vi "welcome.vi"() -> ()   [LabVIEW 2017]
uses:
  GLOBAL/auto.vi
  GLOBAL/all vi close.vi
panel:
  out "first time direct auto":bool
  in  "error in":errorcluster
  in  "EXIT":bool
  in  "PRINTER":bool
  in  "DATA\nHISTORY":bool
  in  "MAIN":bool
  in  "LOGOUT":bool
  in  "USER":bool
  in  "COUNTER":bool
  in  "SETTING":bool
  in  "SHIFT SETTING":bool
  in  "LOGIN":bool
  # "TRACEABILITY"
  # "Powered By- NI Vision, Pune"
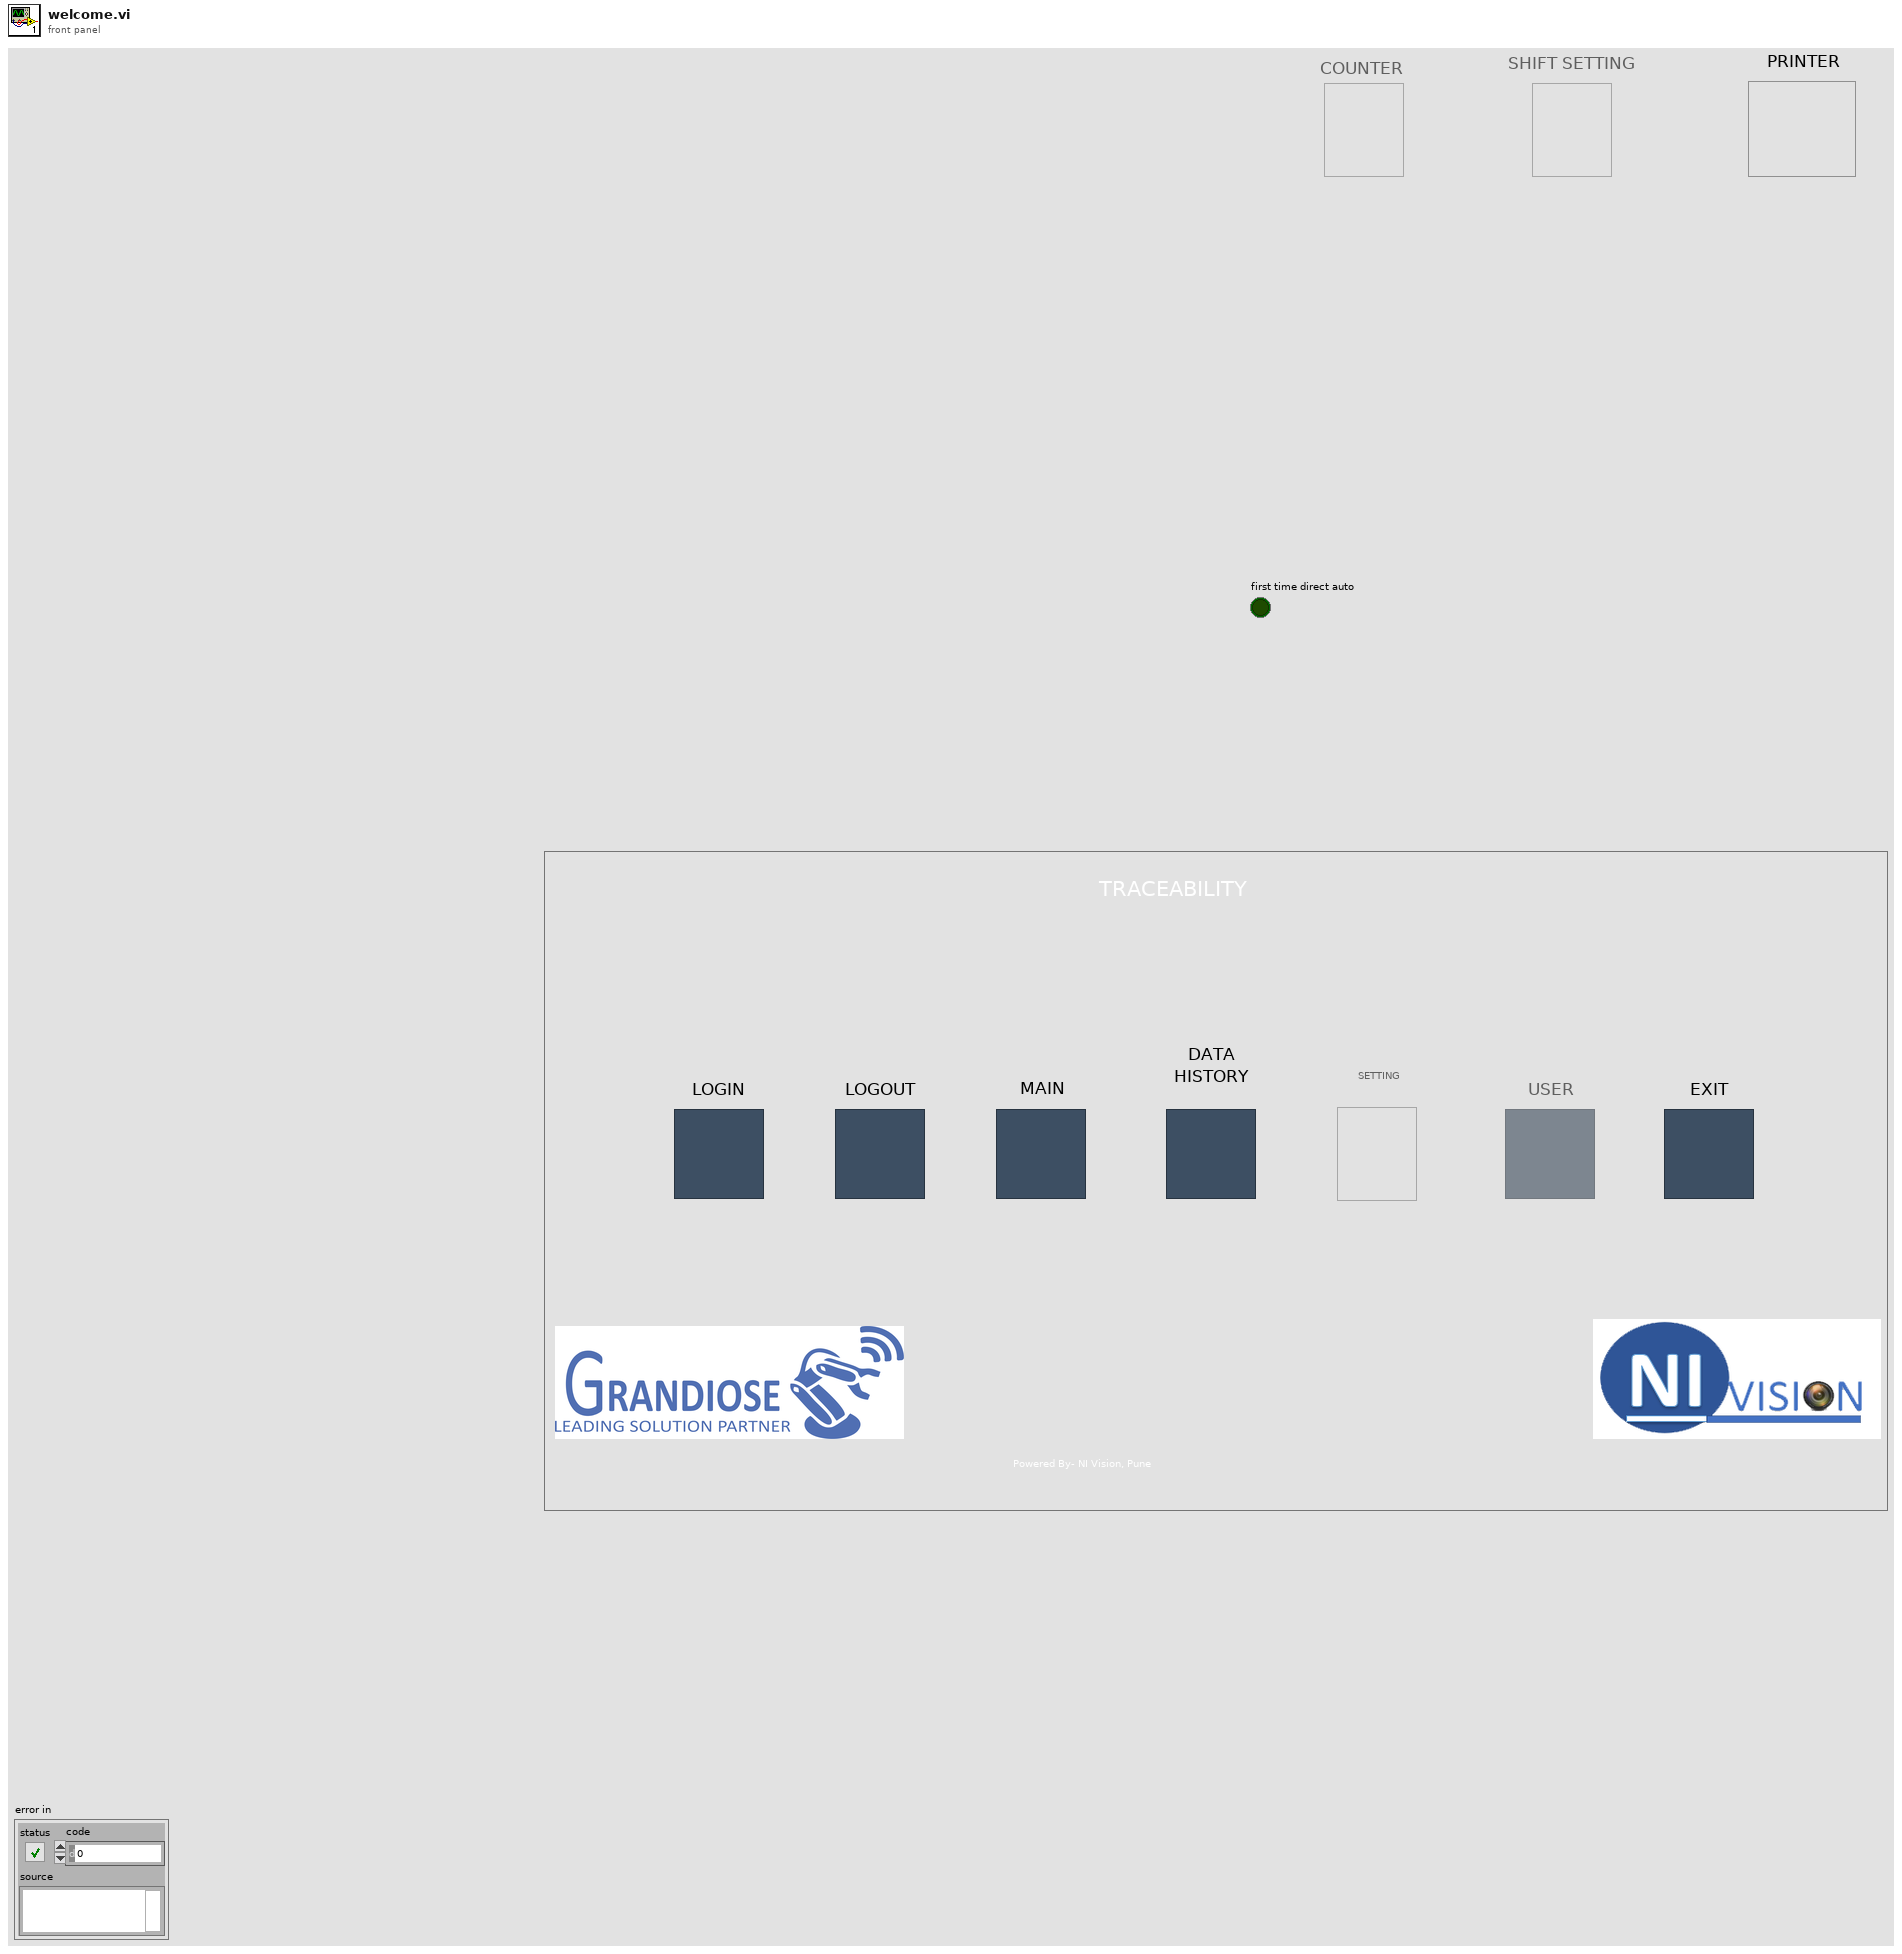
[diagram p1: front panel]
types:
  T1 = enum8{"Enabled", "Disabled", "Disabled and Grayed Out"}
  T2 = enum32{"Invalid", "Standard", "Closed", "Hidden", "Minimized", "Maximized"}
  T3 = enum32{"invalid app kind", "Development System", "Run Time System", "Student Edition", "Embedded LabVIEW", "Evaluation", "Custom"}
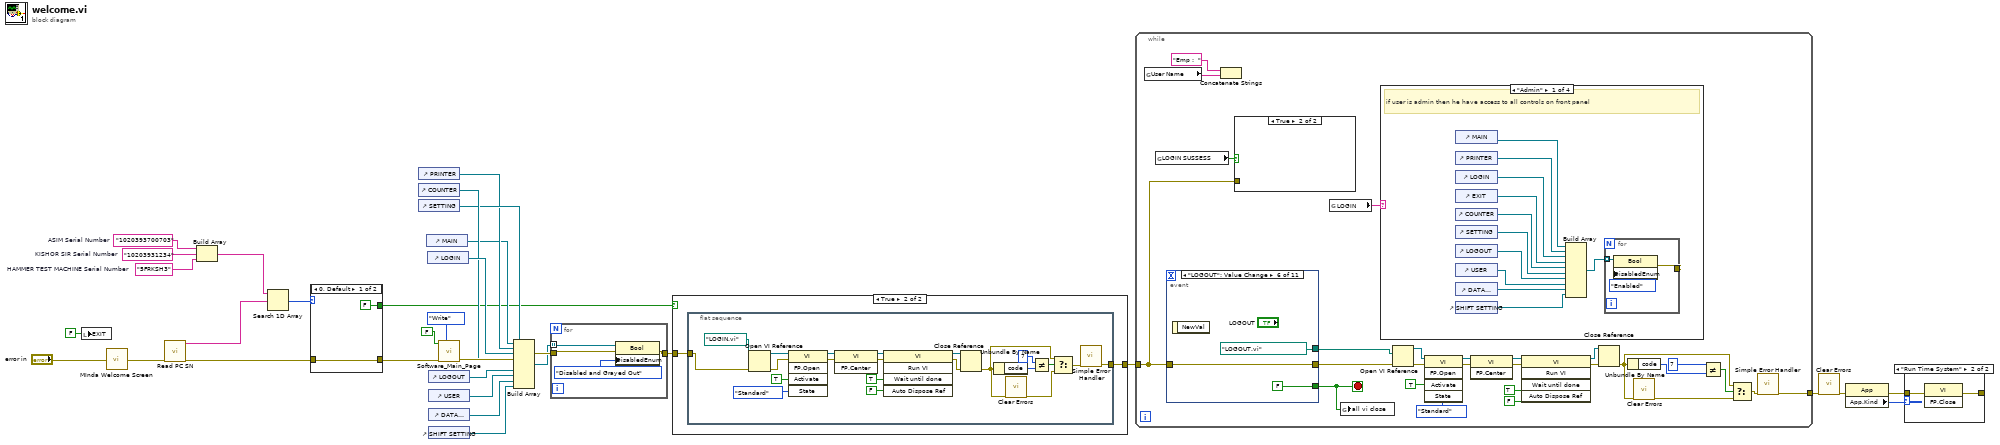
[diagram p0: block diagram]
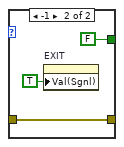
[diagram p3: hidden frame]
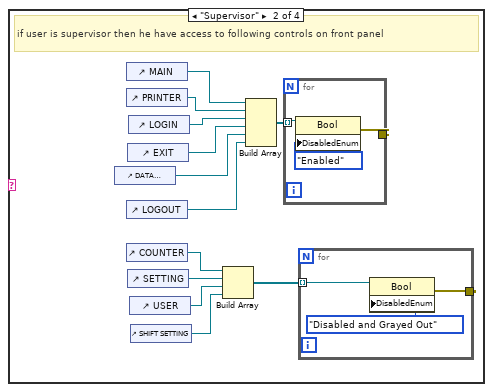
[diagram p6: hidden frame]
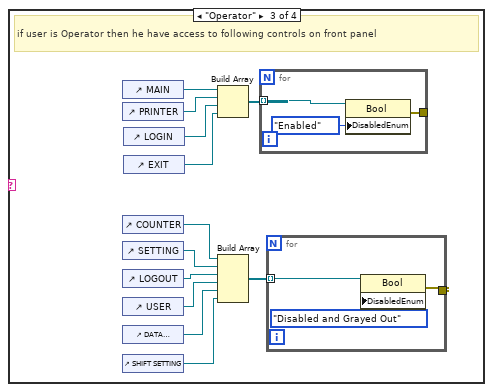
[diagram p7: hidden frame]
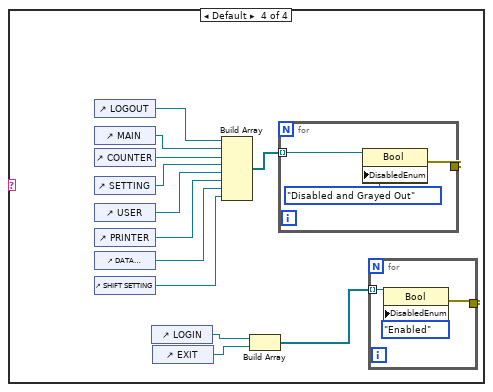
[diagram p8: hidden frame]
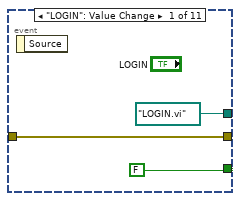
[diagram p9: hidden frame]
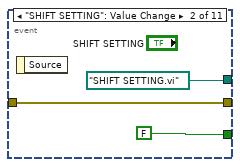
[diagram p10: hidden frame]
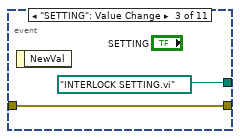
[diagram p11: hidden frame]
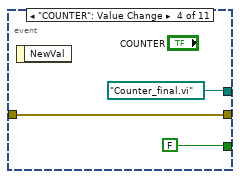
[diagram p12: hidden frame]
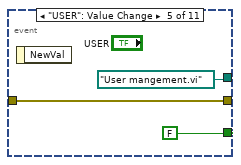
[diagram p13: hidden frame]
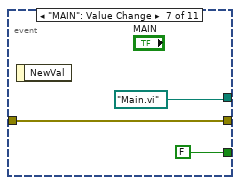
[diagram p14: hidden frame]
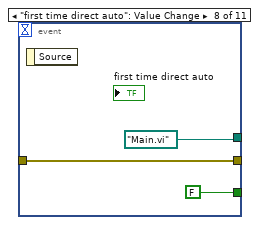
[diagram p15: hidden frame]
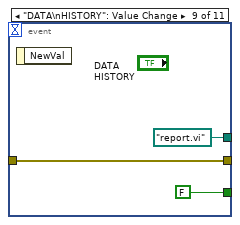
[diagram p16: hidden frame]
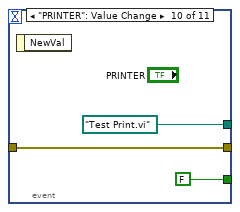
[diagram p17: hidden frame]
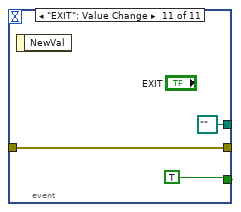
[diagram p18: hidden frame]
diagram:
  w6 = "5FRKSH3"  # HAMMER TEST MACHINE Serial Number
  w7 = "10203931234"  # KISHOR SIR Serial Number
  w8 = "1020393700703"  # ASIM Serial Number
  n1 = local write "EXIT"(FALSE) -> ()
  n2 = call "MInda Welcome Screen.vi"("error in"="error in") -> ("error out"=w10:errorcluster)
  n3 = call "Read PC SN.vi"("error in (no error)"=w10) -> ("error out"=w3:errorcluster, "Serial Number"=w9:string)  [unwired: 9 in]
  n4 = Build Array(w8, w7, w6) -> (w5:string[])
  n5 = Search 1D Array(1D array=w5, element=w9) -> (index of element=w4:i32)  [unwired: 1 in]
  n6 = case shown="0, Default" w4 {
    tunnel: [w33 w35] -> w2
    tunnel: w3 -> [w33 w35]
    tunnel: [FALSE FALSE] -> w1
    frame 0, Default {
    }
    frame -1 {
      n7 = property on="EXIT" class="Bool (strict)"("Val(Sgnl)"=TRUE) -> ()  [unwired: 2 in, 2 out]
    }
  }
  n8 = control-ref of="PRINTER"() -> (w14:refnum<vi>)
  n9 = control-ref of="COUNTER"() -> (w20:refnum<vi>)
  n10 = control-ref of="SETTING"() -> (w19:refnum<vi>)
  n11 = control-ref of="MAIN"() -> (w13:refnum<vi>)
  n12 = control-ref of="LOGIN"() -> (w21:refnum<vi>)
  n13 = control-ref of="LOGOUT"() -> (w18:refnum<vi>)
  n14 = control-ref of="USER"() -> (w17:refnum<vi>)
  n15 = control-ref of="DATA\nHISTORY"() -> (w16:refnum<vi>)
  n16 = control-ref of="SHIFT SETTING"() -> (w15:refnum<vi>)
  n17 = call "Software_Main_Page.vi"("Enum"=enum16{"Read", "Write"}."Write", "error in (no error)"=w2, "Main_Page_in"=FALSE) -> ("error out"=w23:errorcluster)  [unwired: 7 in, 1 out]
  n18 = Build Array(w13, w14, w21, w20, w19, w18, w17, w16, w15) -> (w22:refnum<vi>[])
  n19 = for {
    tunnel: w22 -> [w40] mode=indexing
    tunnel: w23 -> [w38]
    tunnel: [w37] -> w12
    n20 = property class="Bool"(reference=w40, error in=w38, "DisabledEnum"=T1."Disabled and Grayed Out" ("Disabled")) -> (error out=w37:errorcluster)  [unwired: 1 out]
  }
  n21 = case shown="True" w1 {
    tunnel: [w41 w43] -> w30
    tunnel: w12 -> [w41 w42]
    frame False {
    }
    frame True {
      n22 = flat-sequence {
        tunnel: [w45] -> w43
        tunnel: w42 -> [w44]
        frame #0 {
          n23 = Open VI Reference(vi path=path "LOGIN.vi", error in (no error)=w44) -> (vi reference=w52:refnum<vi>, error out=w64:errorcluster)  [unwired: 4 in]
          n24 = invoke class="VI" method="FP.Open"(reference=w52, error in=w64, "Activate"=TRUE ("Activate?"), "State"=T2."Standard") -> (reference out=w63:refnum<vi>, error out=w58:errorcluster)  [unwired: 1 in, 3 out]
          n25 = invoke class="VI" method="FP.Center"(reference=w63, error in=w58) -> (reference out=w59:refnum<vi>, error out=w60:errorcluster)  [unwired: 1 in, 1 out]
          n26 = invoke class="VI" method="Run VI"(reference=w59, error in=w60, "Wait until done"=TRUE ("Wait Until Done"), "Auto Dispose Ref"=FALSE ("Auto Dispose Reference")) -> (reference out=w61:refnum<vi>, error out=w62:errorcluster)  [unwired: 1 in, 3 out]
          n27 = Close Reference(reference=w61, error in (no error)=w62) -> (error out=w53:errorcluster)
          n28 = Unbundle By Name(w53) -> ("code"=w57:i32)
          n29 = call <vilib>:"Clear Errors.vi"("error in (no error)"=w53) -> ("error out"=w55:errorcluster)  [unwired: 5 in, 1 out]
          n30 = Not Equal?(x=7, y=w57) -> (x != y?=w56:bool)
          n31 = Select(t=w53, s=w56, f=w55) -> (s? t:f=w54:errorcluster)
          n32 = call <vilib>:"Simple Error Handler.vi"("error in (no error)"=w54) -> ("error out"=w45:errorcluster)  [unwired: 4 in, 4 out]
        }
      }
    }
  }
  n33 = while {
    tunnel: w30 -> [w67]
    tunnel: [w71] -> w31
    stop <- w69 stop-if-true
    n34 = global read "auto.vi" "User Name"() -> (w66:string)
    n35 = global read "auto.vi" "LOGIN SUSSESS"() -> (w68:bool)
    n36 = event shown="[5] \"LOGOUT\": Value Change" {
      selector: _ -> [_ _ _ _ _ _ _ _ _ _ _]
      dyn-events: _ -> [_ _ _ _ _ _ _ _ _ _ _]
      timeout: _ -> [_ _ _ _ _ _ _ _ _ _ _]
      tunnel: [FALSE FALSE _ FALSE FALSE FALSE FALSE FALSE FALSE FALSE TRUE] -> w69
      tunnel: [path "LOGIN.vi" ("vi path") path "SHIFT SETTING.vi" ("vi path") path "INTERLOCK SETTING.vi" ("vi path") path "Counter_final.vi" ("vi path") path "User mangement.vi" ("vi path") path "LOGOUT.vi" ("vi path") path "Main.vi" ("vi path") path "Main.vi" ("vi path") path "report.vi" ("vi path") path "Test Print.vi" ("vi path") path "" ("vi path")] -> w72
      tunnel: w67 -> [w161 w165 w167 w168 w171 w174 w178 w181 w183 w186 w190]
      tunnel: [w161 w165 w167 w168 w171 w174 w178 w181 w183 w186 w190] -> w73
      event "LOGIN": Value Change {
        n37 = event-data() -> ()  [unwired: 1 in, 1 out]
      }
      event "SHIFT SETTING": Value Change {
        n38 = event-data() -> ()  [unwired: 1 in, 1 out]
      }
      event "SETTING": Value Change {
        n39 = event-data() -> ()  [unwired: 1 in, 1 out]
      }
      event "COUNTER": Value Change {
        n40 = event-data() -> ()  [unwired: 1 in, 1 out]
      }
      event "USER": Value Change {
        n41 = event-data() -> ()  [unwired: 1 in, 1 out]
      }
      event "LOGOUT": Value Change {
        n42 = event-data() -> ()  [unwired: 1 in, 1 out]
      }
      event "MAIN": Value Change {
        n43 = event-data() -> ()  [unwired: 1 in, 1 out]
      }
      event "first time direct auto": Value Change {
        n44 = event-data() -> ()  [unwired: 1 in, 1 out]
      }
      event "DATA\nHISTORY": Value Change {
        n45 = event-data() -> ()  [unwired: 1 in, 1 out]
      }
      event "PRINTER": Value Change {
        n46 = event-data() -> ()  [unwired: 1 in, 1 out]
      }
      event "EXIT": Value Change {
        n47 = event-data() -> ()  [unwired: 1 in, 1 out]
      }
    }
    n48 = Concatenate Strings("Emp :  " ("string"), w66) -> ()  [unwired: 1 out]
    n49 = case shown="True" w68 {
      tunnel: w67 -> [_ _]
      frame False {
      }
      frame True {
      }
    }
    n50 = global read "auto.vi" "LOGIN"() -> (w70:string)
    n51 = global write "all vi close.vi" "all vi close"(w69) -> ()
    n52 = case shown="\"Admin\"" w70 {
      frame "Admin" {
        # "if user is admin then he have access to all controls on front panel"
        n53 = control-ref of="MAIN"() -> (w92:refnum<vi>)
        n54 = control-ref of="PRINTER"() -> (w93:refnum<vi>)
        n55 = control-ref of="LOGIN"() -> (w101:refnum<vi>)
        n56 = control-ref of="EXIT"() -> (w100:refnum<vi>)
        n57 = control-ref of="COUNTER"() -> (w99:refnum<vi>)
        n58 = control-ref of="SETTING"() -> (w98:refnum<vi>)
        n59 = control-ref of="LOGOUT"() -> (w97:refnum<vi>)
        n60 = control-ref of="USER"() -> (w96:refnum<vi>)
        n61 = control-ref of="DATA\nHISTORY"() -> (w95:refnum<vi>)
        n62 = control-ref of="SHIFT SETTING"() -> (w94:refnum<vi>)
        n63 = Build Array(w92, w93, w101, w100, w99, w98, w97, w96, w95, w94) -> (w102:refnum<vi>[])
        n64 = for {
          tunnel: w102 -> [w103] mode=indexing
          tunnel: [w104] -> _
          n65 = property class="Bool"(reference=w103, "DisabledEnum"=T1."Enabled" ("Disabled")) -> (error out=w104:errorcluster)  [unwired: 1 in, 1 out]
        }
      }
      frame "Supervisor" {
        # "if user is supervisor then he have access to following controls on front panel"
        n66 = control-ref of="DATA\nHISTORY"() -> (w113:refnum<vi>)
        n67 = control-ref of="MAIN"() -> (w106:refnum<vi>)
        n68 = control-ref of="PRINTER"() -> (w107:refnum<vi>)
        n69 = control-ref of="LOGOUT"() -> (w112:refnum<vi>)
        n70 = control-ref of="COUNTER"() -> (w111:refnum<vi>)
        n71 = control-ref of="EXIT"() -> (w114:refnum<vi>)
        n72 = control-ref of="SETTING"() -> (w110:refnum<vi>)
        n73 = control-ref of="LOGIN"() -> (w115:refnum<vi>)
        n74 = control-ref of="USER"() -> (w109:refnum<vi>)
        n75 = control-ref of="SHIFT SETTING"() -> (w108:refnum<vi>)
        n76 = Build Array(w111, w110, w109, w108) -> (w116:refnum<vi>[])
        n77 = Build Array(w106, w107, w115, w114, w113, w112) -> (w117:refnum<vi>[])
        n78 = for {
          tunnel: w117 -> [w121] mode=indexing
          tunnel: [w122] -> _
          n79 = property class="Bool"(reference=w121, "DisabledEnum"=T1."Enabled" ("Disabled")) -> (error out=w122:errorcluster)  [unwired: 1 in, 1 out]
        }
        n80 = for {
          tunnel: [w119] -> _
          tunnel: w116 -> [w118] mode=indexing
          n81 = property class="Bool"(reference=w118, "DisabledEnum"=T1."Disabled and Grayed Out" ("Disabled")) -> (error out=w119:errorcluster)  [unwired: 1 in, 1 out]
        }
      }
      frame "Operator" {
        # "if user is Operator then he have access to following controls on front panel"
        n82 = control-ref of="MAIN"() -> (w124:refnum<vi>)
        n83 = control-ref of="PRINTER"() -> (w133:refnum<vi>)
        n84 = control-ref of="COUNTER"() -> (w127:refnum<vi>)
        n85 = control-ref of="SETTING"() -> (w132:refnum<vi>)
        n86 = control-ref of="LOGOUT"() -> (w131:refnum<vi>)
        n87 = control-ref of="USER"() -> (w130:refnum<vi>)
        n88 = control-ref of="DATA\nHISTORY"() -> (w129:refnum<vi>)
        n89 = control-ref of="SHIFT SETTING"() -> (w128:refnum<vi>)
        n90 = control-ref of="LOGIN"() -> (w126:refnum<vi>)
        n91 = control-ref of="EXIT"() -> (w125:refnum<vi>)
        n92 = Build Array(w124, w133, w126, w125) -> (w135:refnum<vi>[])
        n93 = Build Array(w127, w132, w131, w130, w129, w128) -> (w134:refnum<vi>[])
        n94 = for {
          tunnel: w135 -> [w141] mode=indexing
          tunnel: [w139] -> _
          n95 = property class="Bool"(reference=w141, "DisabledEnum"=T1."Enabled" ("Disabled")) -> (error out=w139:errorcluster)  [unwired: 1 in, 1 out]
        }
        n96 = for {
          tunnel: w134 -> [w138] mode=indexing
          tunnel: [w136] -> _
          n97 = property class="Bool"(reference=w138, "DisabledEnum"=T1."Disabled and Grayed Out" ("Disabled")) -> (error out=w136:errorcluster)  [unwired: 1 in, 1 out]
        }
      }
      frame Default {
        n98 = control-ref of="LOGOUT"() -> (w146:refnum<vi>)
        n99 = control-ref of="MAIN"() -> (w145:refnum<vi>)
        n100 = control-ref of="COUNTER"() -> (w147:refnum<vi>)
        n101 = control-ref of="SETTING"() -> (w148:refnum<vi>)
        n102 = control-ref of="USER"() -> (w149:refnum<vi>)
        n103 = control-ref of="PRINTER"() -> (w150:refnum<vi>)
        n104 = control-ref of="DATA\nHISTORY"() -> (w151:refnum<vi>)
        n105 = control-ref of="SHIFT SETTING"() -> (w152:refnum<vi>)
        n106 = control-ref of="LOGIN"() -> (w142:refnum<vi>)
        n107 = control-ref of="EXIT"() -> (w144:refnum<vi>)
        n108 = Build Array(w146, w145, w147, w148, w149, w150, w151, w152) -> (w153:refnum<vi>[])
        n109 = Build Array(w142, w144) -> (w143:refnum<vi>[])
        n110 = for {
          tunnel: w153 -> [w157] mode=indexing
          tunnel: [w158] -> _
          n111 = property class="Bool"(reference=w157, "DisabledEnum"=T1."Disabled and Grayed Out" ("Disabled")) -> (error out=w158:errorcluster)  [unwired: 1 in, 1 out]
        }
        n112 = for {
          tunnel: w143 -> [w154] mode=indexing
          tunnel: [w155] -> _
          n113 = property class="Bool"(reference=w154, "DisabledEnum"=T1."Enabled" ("Disabled")) -> (error out=w155:errorcluster)  [unwired: 1 in, 1 out]
        }
      }
    }
    n114 = Open VI Reference(vi path=w72, error in (no error)=w73) -> (vi reference=w91:refnum<vi>, error out=w80:errorcluster)  [unwired: 4 in]
    n115 = invoke class="VI" method="FP.Open"(reference=w91, error in=w80, "Activate"=TRUE ("Activate?"), "State"=T2."Standard") -> (reference out=w81:refnum<vi>, error out=w86:errorcluster)  [unwired: 1 in, 3 out]
    n116 = invoke class="VI" method="FP.Center"(reference=w81, error in=w86) -> (reference out=w85:refnum<vi>, error out=w84:errorcluster)  [unwired: 1 in, 1 out]
    n117 = invoke class="VI" method="Run VI"(reference=w85, error in=w84, "Wait until done"=TRUE ("Wait Until Done"), "Auto Dispose Ref"=FALSE ("Auto Dispose Reference")) -> (reference out=w83:refnum<vi>, error out=w82:errorcluster)  [unwired: 1 in, 3 out]
    n118 = Close Reference(reference=w83, error in (no error)=w82) -> (error out=w79:errorcluster)
    n119 = Unbundle By Name(w79) -> ("code"=w87:i32)
    n120 = call <vilib>:"Clear Errors.vi"("error in (no error)"=w79) -> ("error out"=w89:errorcluster)  [unwired: 5 in, 1 out]
    n121 = Not Equal?(x=7, y=w87) -> (x != y?=w88:bool)
    n122 = Select(t=w79, s=w88, f=w89) -> (s? t:f=w90:errorcluster)
    n123 = call <vilib>:"Simple Error Handler.vi"("error in (no error)"=w90) -> ("error out"=w71:errorcluster)  [unwired: 4 in, 4 out]
  }
  n124 = call <vilib>:"Clear Errors.vi"("error in (no error)"=w31) -> ("error out"=w27:errorcluster)  [unwired: 5 in, 1 out]
  n125 = property class="App"(error in=w27) -> (error out=w28:errorcluster, "App.Kind"=w29:T3)  [unwired: 1 in, 1 out]
  n126 = case shown="\"Run Time System\"" w29 {
    tunnel: w28 -> [w192 w194]
    tunnel: [w192 w193] -> _
    frame Default {
    }
    frame "Run Time System" {
      n127 = invoke class="VI" method="FP.Close"(error in=w194) -> (error out=w193:errorcluster)  [unwired: 2 in, 2 out]
    }
  }
